vi "Debug_Convert_Data_to_String.vi"(8 "error in (no error)":errorcluster, 11 "AB_Source in":refnum<class "AB_Source.lvclass">) -> (0 "error out":errorcluster, 1 "classData":string, 2 "sourceType":string, 3 "AB_Source out":refnum<class "AB_Source.lvclass">)   [LabVIEW 2020, in "AB_Source.lvclass"]
uses:
  <vilib>/AppBuilder/AB_Classes/Source/AB_Source.lvclass
  <vilib>/AppBuilder/AB_Classes/Source/AB_Source.lvclass/AB_Source.ctl
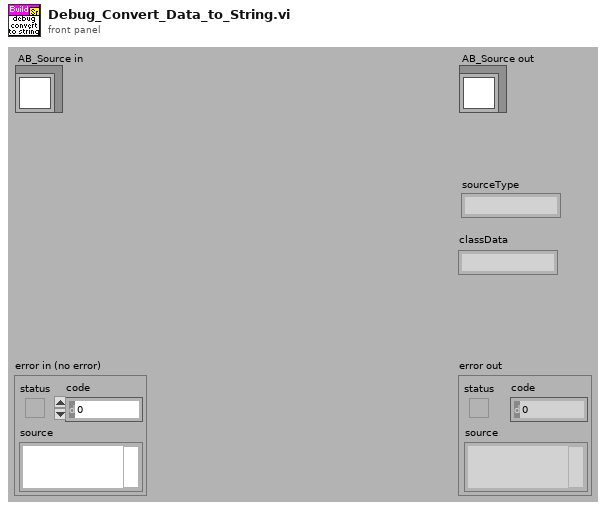
[diagram p1: front panel]
types:
  T1 = typedef "AB_Source_Inclusion.ctl" = enum16{"IncludeIfReferenced", "Include", "Exclude", "TopLevel"}
  T2 = typedef "AB_Source_Properties.ctl" = cluster{"sourcePropertyType":T3, "value":variant}
  T3 = typedef "AB_Source_Property_Type.ctl" = enum16{"Remove block diagram", "Remove front panel", "Password", "Window has title bar", "Show menu bar", "Show vertical scroll bar", "Show horizontal scroll bar", "Show toolbar", "Show Abort button", "Show fp when called", "Window behavior", "Allow user to close window", "Window run-time position", "Run when opened", "Allow debugging", "Auto error handling", "Generate guard code", "Use stack variables", "Expression folding", "Integer only", "Inline subVI"}
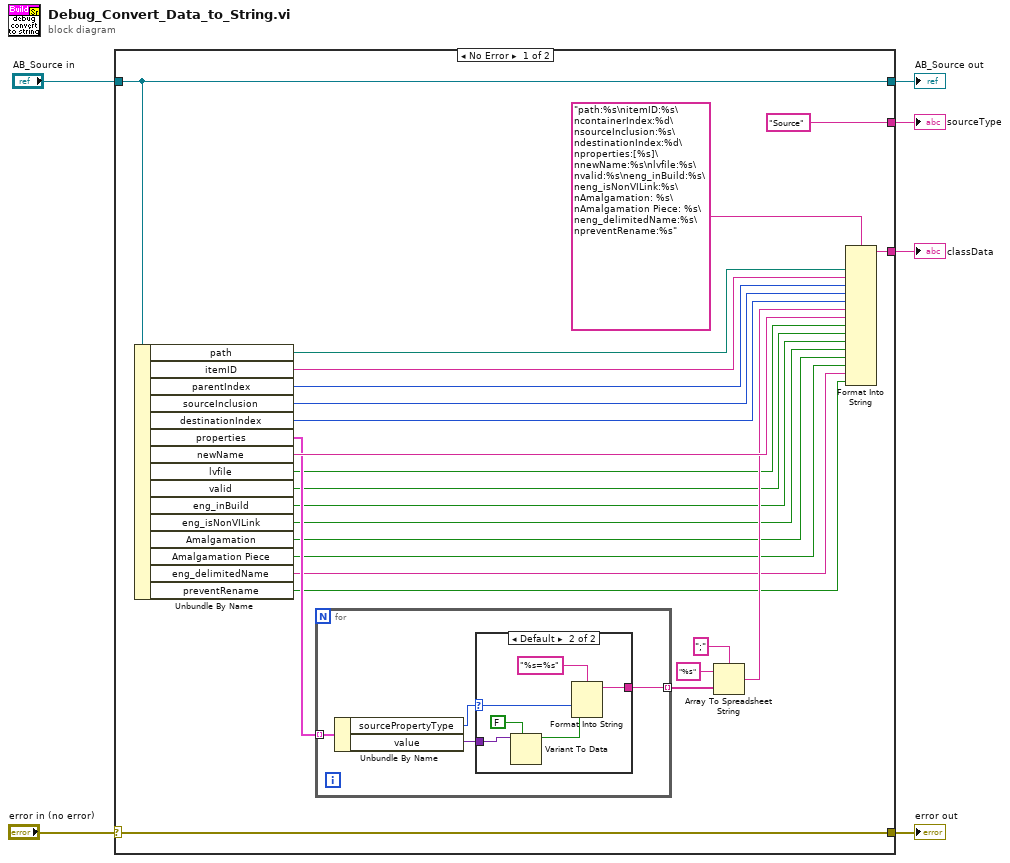
[diagram p0: block diagram]
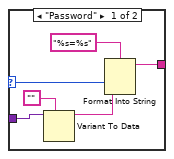
[diagram p2: hidden frame]
diagram:
  n1 = case shown="No Error" "error in (no error)" {
    selector: "error in (no error)" -> [w30 w48]
    tunnel: [w30 w48] -> w5
    tunnel: [w29 w47] -> w3
    tunnel: "AB_Source in" -> [w29 w47]
    tunnel: [w21 _] -> w2
    tunnel: ["Source" _] -> w1
    frame No Error {
      n2 = Unbundle By Name(w29) -> ("path"=w27:path, "itemID"=w26:string, "parentIndex"=w25:i32, "sourceInclusion"=w24:T1, "destinationIndex"=w23:i32, "properties"=w20:T2[], "newName"=w22:string, "lvfile"=w13:bool, "valid"=w12:bool, "eng_inBuild"=w14:bool, "eng_isNonVILink"=w11:bool, "Amalgamation"=w10:bool, "Amalgamation Piece"=w9:bool, "eng_delimitedName"=w8:string, "preventRename"=w7:bool)
      n3 = for {
        tunnel: w20 -> [w34] mode=indexing
        tunnel: [w31] -> w17 mode=indexing
        n4 = Unbundle By Name(w34) -> ("sourcePropertyType"=w33:T3, "value"=w32:variant)
        n5 = case shown="Default" w33 {
          selector: w33 -> [w36 w43]
          tunnel: w32 -> [w40 w46]
          tunnel: [w37 w44] -> w31
          frame "Password" {
            n6 = Variant To Data(type="", Variant=w40) -> (data=w35:string)  [unwired: 1 in, 1 out]
            n7 = Format Into String(format string="%s=%s", w36, w35) -> (resulting string=w37:string)  [unwired: 2 in, 1 out]
          }
          frame Default {
            n8 = Variant To Data(type=FALSE, Variant=w46) -> (data=w42:bool)  [unwired: 1 in, 1 out]
            n9 = Format Into String(format string="%s=%s", w43, w42) -> (resulting string=w44:string)  [unwired: 2 in, 1 out]
          }
        }
      }
      n10 = Array To Spreadsheet String(delimiter (Tab)=";", array=w17, 3:"%s" ("format string")) -> (spreadsheet string=w16:string)
      n11 = Format Into String(format string="path:%s\nitemID:%s\ncontainerIndex:%d\nsourceInclusion:%s\ndestinationIndex:%d\nproperties:[%s]\nnewName:%s\nlvfile:%s\nvalid:%s\neng_inBuild:%s\neng_isNonVILink:%s\nAmalgamation: %s\nAmalgamation Piece: %s\neng_delimitedName:%s\npreventRename:%s", w27, w26, w25, w24, w23, w16, w22, w13, w12, w14, w11, w10, w9, w8, w7) -> (resulting string=w21:string)  [unwired: 2 in, 1 out]
    }
    frame Error {
    }
  }
  "error out" <- w5
  "AB_Source out" <- w3
  "classData" <- w2
  "sourceType" <- w1
